vi "open_usb_port.vi"(8 "error in (no error)":errorcluster) -> (0 "error out":errorcluster, 1 "failstring":string, 2 "opened":bool, 3 "device_handle":i32)   [LabVIEW 2014, in "Dali_usb.lvlib"]
uses:
  Dali_usb.lvlib
  dll/DaliBusAccess.dll
panel:
  out "hWnd":i32
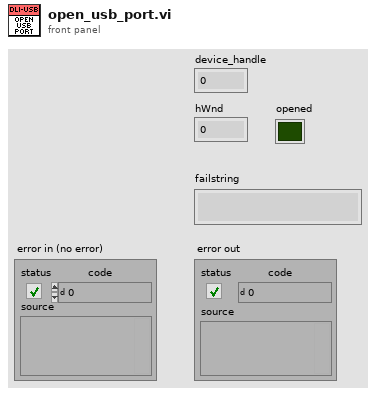
[diagram p1: front panel]
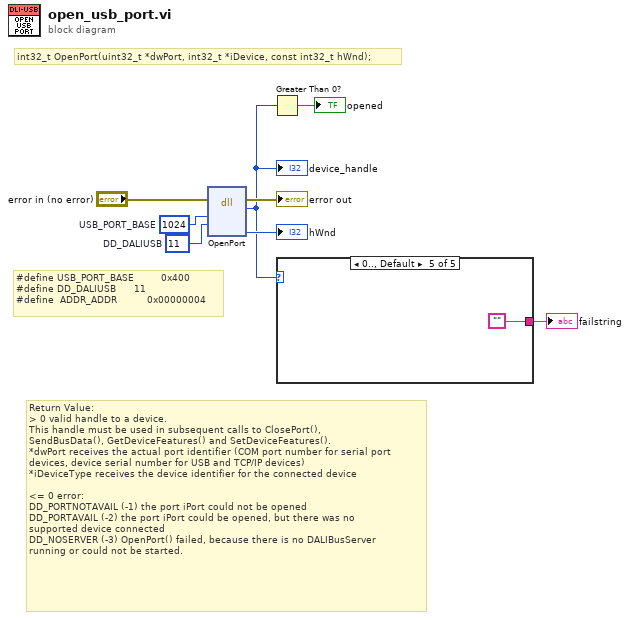
[diagram p0: block diagram]
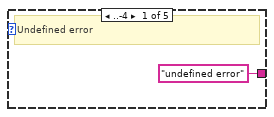
[diagram p2: hidden frame]
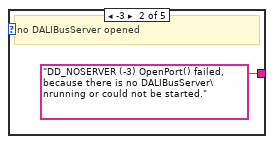
[diagram p3: hidden frame]
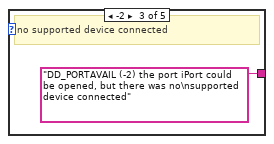
[diagram p4: hidden frame]
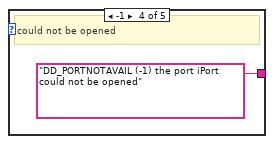
[diagram p5: hidden frame]
diagram:
  w8 = 11  # DD_DALIUSB
  w7 = u32 1024  # USB_PORT_BASE
  # "#define USB_PORT_BASE\t\t       0x400 \n#define DD_DALIUSB\t\t    11\n#define  ADDR_ADDR          0x00000004"
  # "Return Value:\n> 0 valid handle to a device. \nThis handle must be used in subsequent calls to ClosePort(),\nSendBusData(), GetDeviceFeatures() and SetDeviceFeatures().\n*dwPort receives the actual port identifier (COM port number for serial port\ndevices, device serial number for USB and TCP/IP devices)\n*iDeviceType receives the device identifier for the connected device\n\n<= 0 error:\nDD_PORTNOTAVAIL (-1) the port iPort could not be opened\nDD_PORTAVAIL (-2) the port iPort could be opened, but there was no\nsupported device connected\nDD_NOSERVER (-3) OpenPort() failed, because there is no DALIBusServer\nrunning or could not be started."
  # "int32_t OpenPort(uint32_t *dwPort, int32_t *iDevice, const int32_t hWnd);"
  n1 = dll-call lib="C:/LTS/app-tde-luminaires/SourceCode/Instruments/Driver_interaction/Dali_usb/Vendor/dll/DaliBusAccess.dll" fn="OpenPort"(error in="error in (no error)", "dwPort"=w7, "iDevice"=w8) -> (error out=→"error out":errorcluster, "return type"=w3:i32, "hWnd"=→"hWnd":i32)  [unwired: 5 in, 1 out]
  "device_handle" <- w3
  n2 = Greater Than 0?(x=w3) -> (x > 0?=→"opened":bool)
  n3 = case shown="0.., Default" w3 {
    tunnel: ["undefined error" "DD_NOSERVER (-3) OpenPort() failed, because there is no DALIBusServer\nrunning or could not be started." "DD_PORTAVAIL (-2) the port iPort could be opened, but there was no\nsupported device connected" "DD_PORTNOTAVAIL (-1) the port iPort could not be opened" ""] -> w1
    frame ..-4 {
      # "Undefined error"
    }
    frame -3 {
      # "no DALIBusServer opened"
    }
    frame -2 {
      # "no supported device connected"
    }
    frame -1 {
      # "could not be opened"
    }
    frame 0.., Default {
    }
  }
  "failstring" <- w1
